vi "BeamWidthCalc.vi"(8 "Not dB?":bool, 9 "dB width pt":dbl, 10 "y values":dbl[](array[numeric]), 11 "x values":dbl[](array[numeric])) -> (3 "Output variables":T1, 4 "Freqs":dbl[](array[numeric]), 7 "Plot Values":cluster{dbl[], dbl[]})   [LabVIEW 2022 SP3]
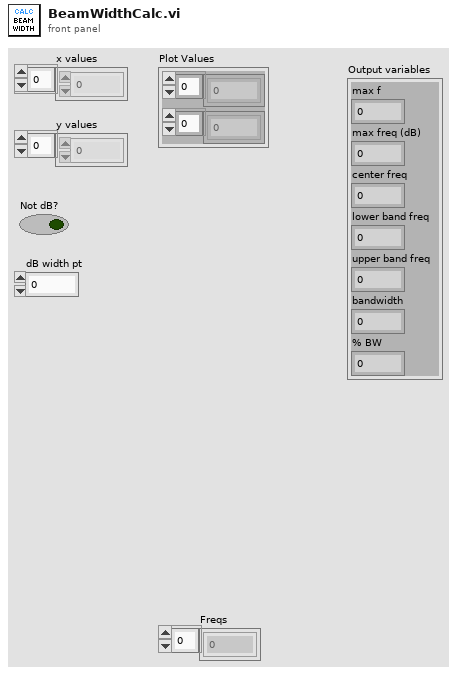
[diagram p1: front panel]
types:
  T1 = cluster{"max f":sgl, "max freq (dB)":sgl, "center freq":sgl, "lower band freq":sgl, "upper band freq":sgl, "bandwidth":sgl, "% BW":dbl}
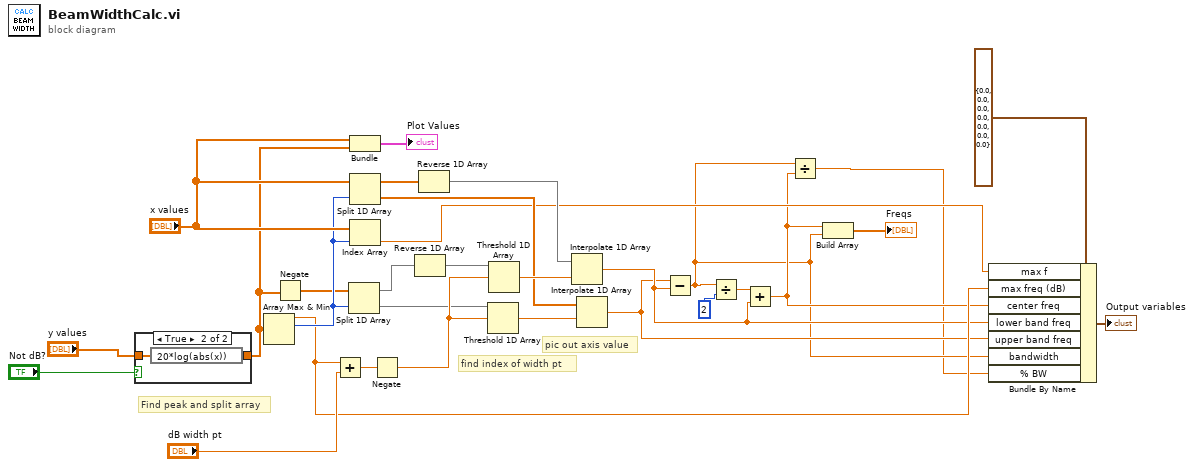
[diagram p0: block diagram]
diagram:
  # "Find peak and split array"
  # "find index of width pt"
  # "pic out axis value"
  n1 = case shown="True" "Not dB?" {
    tunnel: "y values" -> [w31 w33]
    tunnel: [w31 w32] -> w28
    frame False {
    }
    frame True {
      n2 = expression code="20*log(abs(x))"(w33) -> (w32:dbl[])
    }
  }
  n3 = Array Max & Min(array=w28) -> (max value=w7:dbl, max index (indices)=w12:i32)  [unwired: 2 out]
  n4 = Negate(x=w28) -> (-x=w10:dbl[])
  n5 = Add(x=w7, y="dB width pt") -> (x+y=w11:dbl)
  n6 = Split 1D Array(array=w10, index=w12) -> (first subarray=w13:dbl[], second subarray=w15:dbl[])
  n7 = Bundle("x values"="x values", "y values"=w28) -> (→"Plot Values":cluster{"x values":dbl[], "y values":dbl[]})  [unwired: 1 out]
  n8 = Split 1D Array(array="x values", index=w12) -> (first subarray=w16:dbl[], second subarray=w18:dbl[])
  n9 = Index Array(array="x values", index=w12) -> (element=w8:dbl)
  n10 = Negate(x=w11) -> (-x=w23:dbl)
  n11 = Reverse 1D Array(array=w13) -> (reversed array=w14:dbl[])
  n12 = Reverse 1D Array(array=w16) -> (reversed array=w17:dbl[])
  n13 = Threshold 1D Array(2:w23, 3:w15) -> (0:w20:dbl)  [unwired: 1 out]
  n14 = Threshold 1D Array(2:w23, 3:w14) -> (0:w19:dbl)  [unwired: 1 out]
  n15 = Interpolate 1D Array(1:w19, 2:w17) -> (0:w5:dbl)
  n16 = Interpolate 1D Array(1:w20, 2:w18) -> (0:w4:dbl)
  n17 = Subtract(x=w4, y=w5) -> (x-y=w3:dbl)
  n18 = Divide(x=w3, y=2) -> (x/y=w22:dbl)
  n19 = Add(x=w22, y=w5) -> (x+y=w6:dbl)
  n20 = Divide(x=w3, y=w6) -> (x/y=w2:dbl)
  n21 = Build Array(w6, w3) -> (→"Freqs":dbl[])
  n22 = Bundle By Name(cluster=T1 {"max f"=0.0, "max freq (dB)"=0.0, "center freq"=0.0, "lower band freq"=0.0, "upper band freq"=0.0, "bandwidth"=0.0, "% BW"=0.0} ("Output variables"), "max f"=w8, "max freq (dB)"=w7, "center freq"=w6, "lower band freq"=w5, "upper band freq"=w4, "bandwidth"=w3, "% BW"=w2) -> (→"Output variables":T1)
